vi "xively_average_Wh.vi"(1 "Power":dbl, 2 "queue out":refnum<queue>) -> (0 "DSSC1*":dbl)   [LabVIEW 2012]
panel:
  out "# elements in queue":i32
  in  "stop":bool
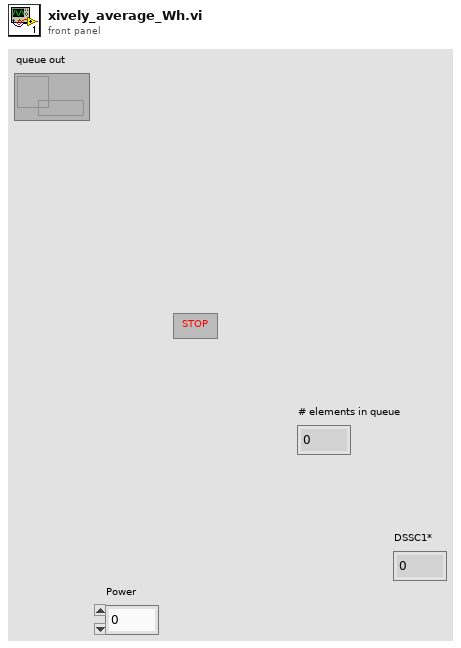
[diagram p1: front panel]
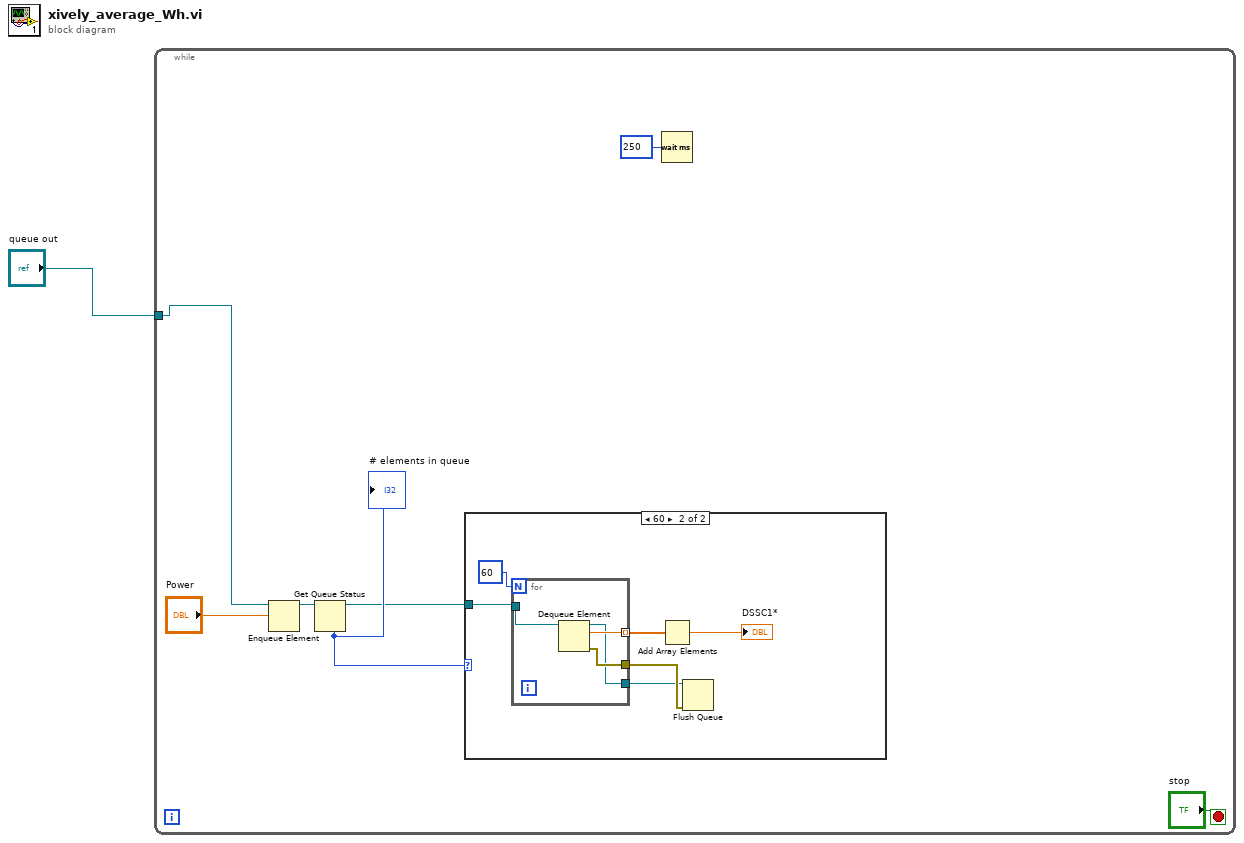
[diagram p0: block diagram]
diagram:
  n1 = while {
    tunnel: "queue out" -> [w7]
    stop <- "stop" stop-if-true
    n2 = Enqueue Element(queue=w7, element="Power") -> (queue out=w4:refnum<queue>)  [unwired: 2 in, 2 out]
    n3 = Get Queue Status(queue=w4) -> (queue out=w3:refnum<queue>, # elements in queue=w5:i32)  [unwired: 2 in, 6 out]
    "# elements in queue" <- w5
    n4 = case shown="60" w5 {
      tunnel: w3 -> [_ w14]
      frame 0, Default {
      }
      frame 60 {
        n5 = for {
          N: 60 -> [_]
          tunnel: w14 -> [w18]
          tunnel: [w17] -> w12 mode=indexing
          tunnel: [w16] -> w11
          tunnel: [w15] -> w10
          n6 = Dequeue Element(queue=w18) -> (queue out=w15:refnum<queue>, element=w17:dbl, error out=w16:errorcluster)  [unwired: 2 in, 1 out]
        }
        n7 = Add Array Elements(numeric array=w12) -> (sum=→"DSSC1*":dbl)
        n8 = Flush Queue(queue=w10, error in (no error)=w11) -> ()  [unwired: 3 out]
      }
    }
    n9 = Wait (ms)(milliseconds to wait=u32 250) -> ()  [unwired: 1 out]
  }
